vi "Drive Straight PID.vi"(5 "Angle Offset":dbl, 6 "Iteration":i32, 7 "target distance":dbl, 8 "Period (ms)":i64=10) -> (1 "Complete?":bool, 2 "Right Axis":dbl, 3 "Left Axis":dbl)   [LabVIEW 2017]
uses:
  Odometry/Typedef/Odometry.ctl
  <vilib>/addons/control/pid/pid.llb/PID Output Rate Limiter (DBL).vi
  <vilib>/addons/control/pid/NI_PID_pid.lvlib
panel:
  in  "Odometry":T1
  in  "output rate":dbl=80.0 format="%.2f"
  in  "Gyro PIDF":cluster{"Kp":dbl, "Ki":dbl, "Kd":dbl, "Kf":dbl}={"Kp"=0.05, "Ki"=0.0, "Kd"=0.0, "Kf"=0.0} {"Kf" format="%.3f"; "Kd" format="%.3f"; "Ki" format="%.3f"; "Kp" format="%.3f"}
  in  "PIDF":cluster{"Kp":dbl, "Ki":dbl, "Kd":dbl, "Kf":dbl}={"Kp"=0.02, "Ki"=0.0, "Kd"=0.045, "Kf"=0.0} {"Kf" format="%.3f"; "Kd" format="%.3f"; "Ki" format="%.3f"; "Kp" format="%.3f"}
  in  "i Zone":dbl=12.0 format="%.2f"
  in  "output range":cluster{"output high":dbl, "output low":dbl}={"output high"=1.0, "output low"=-1.0} {"output low" format="%.2f"; "output high" format="%.2f"}
  out "Waveform Chart 2":cluster{dbl, dbl}(graph)={-50.0, -50.00778875}
  out "Gyro Output":dbl(graph)=0.02713616249999992
  out "mean":dbl=0.00016497888749945157 format="%0.2f"
  in  "threshold":dbl=0.008
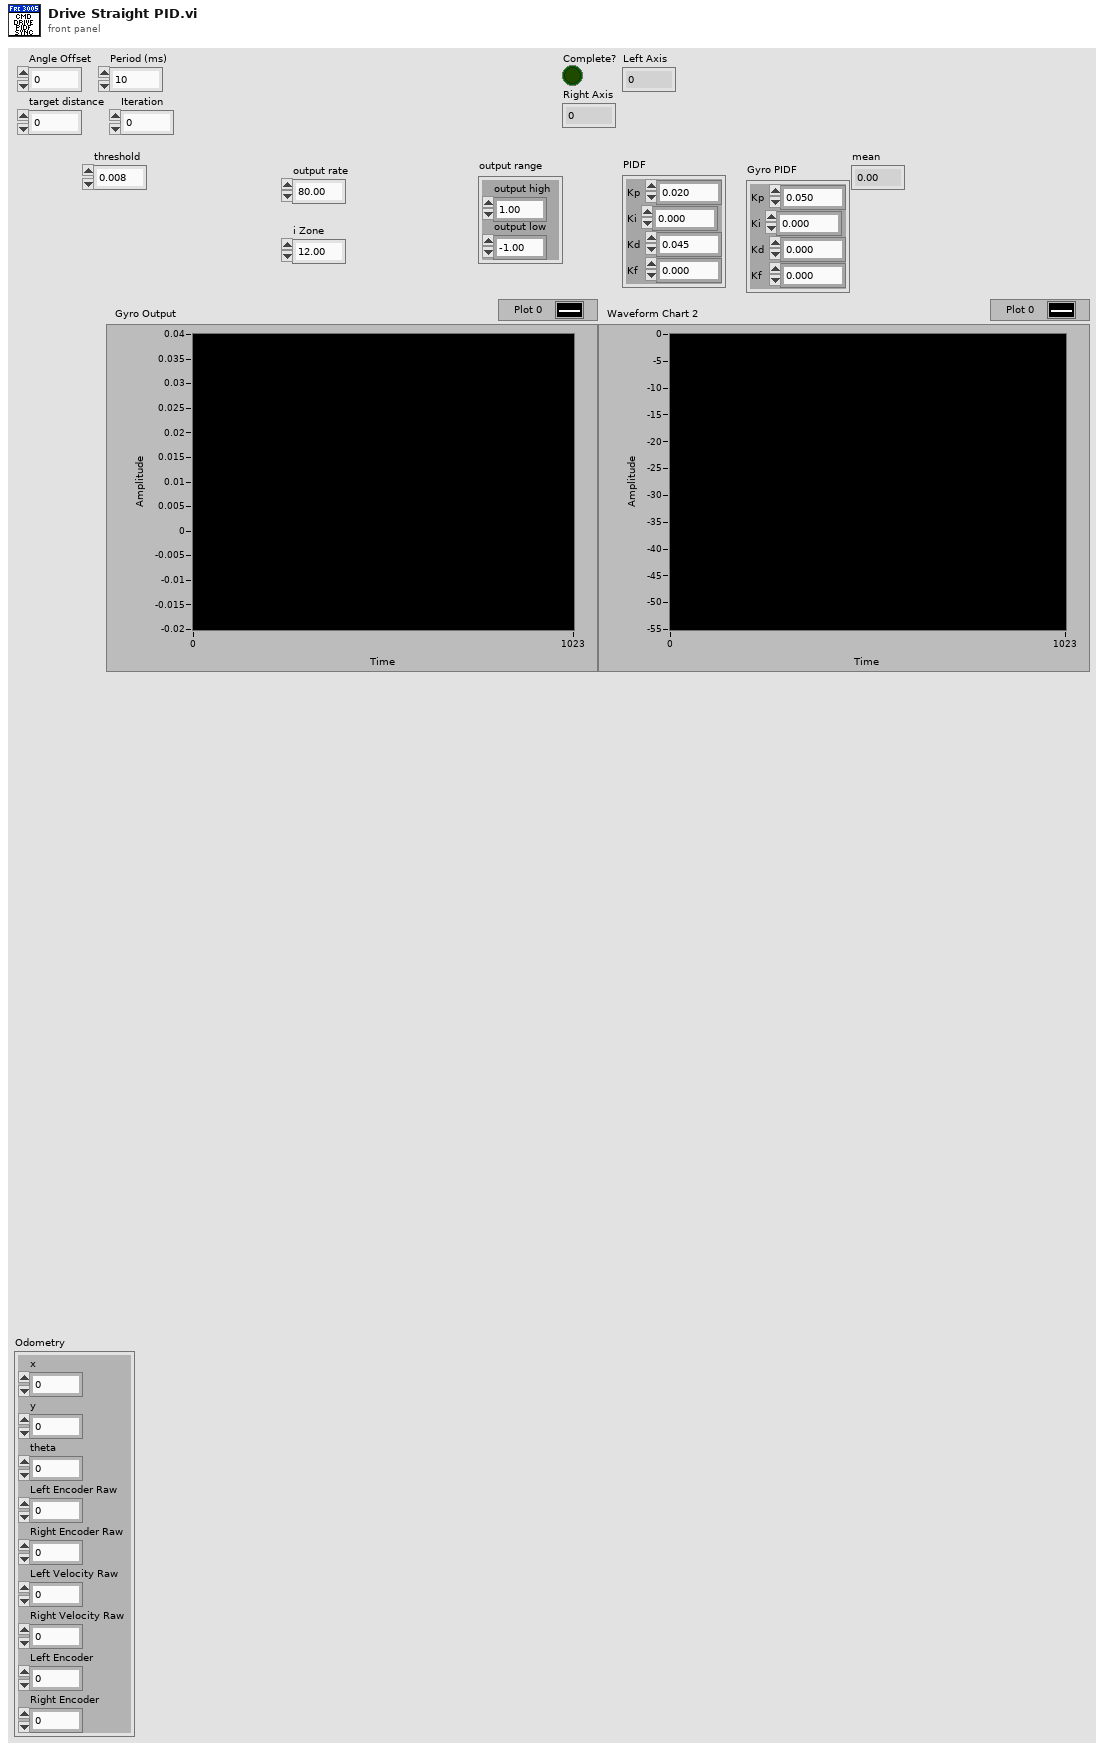
[diagram p1: front panel]
types:
  T1 = typedef "Odometry.ctl" = cluster{"x":dbl, "y":dbl, "theta":dbl, "Left Encoder Raw":i32, "Right Encoder Raw":i32, "Left Velocity Raw":i32, "Right Velocity Raw":i32, "Left Encoder":dbl, "Right Encoder":dbl}
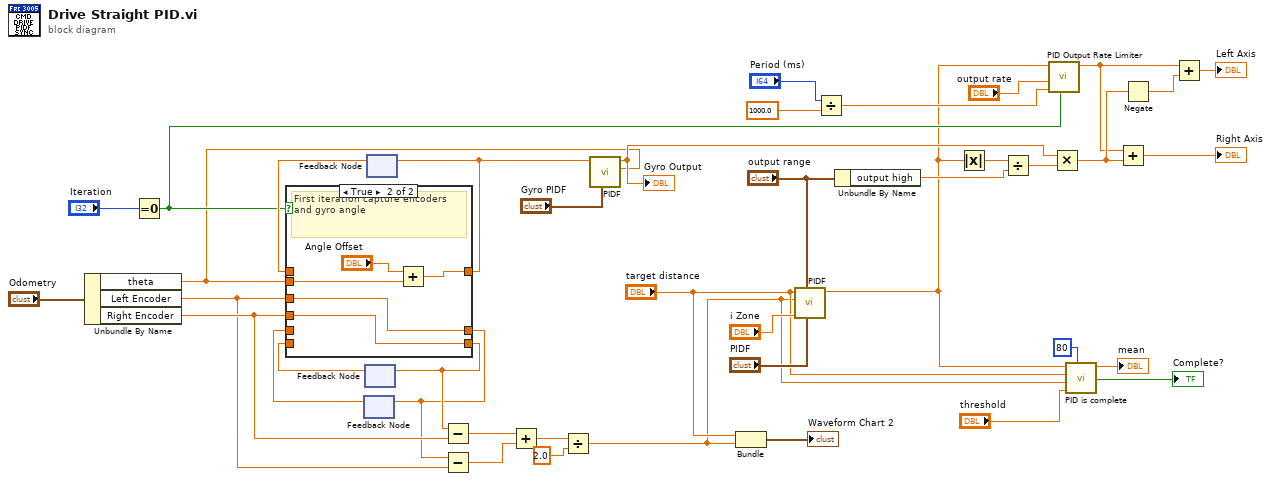
[diagram p0: block diagram]
diagram:
  n1 = Unbundle By Name("Odometry") -> ("theta"=w9:dbl, "Left Encoder"=w3:dbl, "Right Encoder"=w5:dbl)
  n2 = Equal To 0?(x="Iteration") -> (x = 0?=w19:bool)
  n3 = feedback #1() -> (w7:dbl)  [unwired: 1 in]
  n4 = feedback #2() -> (w8:dbl)  [unwired: 1 in]
  n5 = feedback #3() -> (w21:dbl)  [unwired: 1 in]
  n6 = case shown="True" w19 {
    tunnel: [w44 w48] -> w22
    tunnel: w21 -> [w44 _]
    tunnel: w9 -> [_ w47]
    tunnel: w3 -> [_ w45]
    tunnel: w5 -> [_ w46]
    tunnel: [w43 w46] -> w6
    tunnel: [w42 w45] -> w4
    tunnel: w8 -> [w43 _]
    tunnel: w7 -> [w42 _]
    frame False {
    }
    frame True {
      # "First iteration capture encoders and gyro angle"
      n7 = Add(x="Angle Offset", y=w47) -> (x+y=w48:dbl)
    }
  }
  n8 = feedback-in #1(w4) -> ()
  n9 = feedback-in #2(w6) -> ()
  n10 = feedback-in #3(w22) -> ()
  n11 = Subtract(x=w6, y=w5) -> (x-y=w2:dbl)
  n12 = Subtract(x=w4, y=w3) -> (x-y=w1:dbl)
  n13 = Add(x=w2, y=w1) -> (x+y=w41:dbl)
  n14 = Divide(x=w41, y=2.0) -> (x/y=w11:dbl)
  n15 = call "PIDF.vi"("PIDF gains"="Gyro PIDF", "process variable"=w9, "setpoint"=w22) -> ("output"=w32:dbl)  [unwired: 6 in, 2 out]
  "Gyro Output" <- w32
  n16 = Bundle("target distance"="target distance", w11) -> (→"Waveform Chart 2":cluster{"target distance":dbl, dbl})  [unwired: 1 in]
  n17 = call "PIDF.vi"("PIDF gains"="PIDF", "output range"="output range", "i Zone"="i Zone", "process variable"=w11, "setpoint"="target distance") -> ("output"=w15:dbl)  [unwired: 4 in, 2 out]
  n18 = Divide(x="Period (ms)", y=1000.0) -> (x/y=w37:dbl)
  n19 = Unbundle By Name("output range") -> ("output high"=w28:dbl)
  n20 = Absolute Value(x=w15) -> (abs(x)=w14:dbl)
  n21 = Divide(x=w14, y=w28) -> (x/y=w27:dbl)
  n22 = call-poly <vilib>:"PID Output Rate Limiter.vi"("reinitialize? (F)"=w19, "dt (s)"=w37, "output rate (EGU/min)"="output rate", "input (controller output)"=w15) -> ("output"=w24:dbl)  [unwired: 4 in, 1 out]
  n23 = Multiply(x=w32, y=w27) -> (x*y=w30:dbl)
  n24 = call "PID is complete.vi"("sample length"=80, "threshold"="threshold", "process variable"=w11, "setpoint"="target distance", "PID Output"=w15) -> ("PID is Done?"=→"Complete?":bool, "mean"=→"mean":dbl)  [unwired: 5 in]
  n25 = Add(x=w24, y=w30) -> (x+y=→"Right Axis":dbl)
  n26 = Negate(x=w30) -> (-x=w31:dbl)
  n27 = Add(x=w24, y=w31) -> (x+y=→"Left Axis":dbl)
